vi "Send State.vi"(8 "entrée d'erreur (pas d'erreur)":errorcluster, 11 "State":T1(ring)) -> (0 "sortie d'erreur":errorcluster)   [LabVIEW 2020, in "Library Core.lvlib" / "Actor_EventStart.lvlib" / "Actor_EventStart.lvclass"]
uses:
  Actor_EventStart.lvclass
  Commun VI/TypeDef/Variable Printable.ctl
  Actor_EventStart Messages/Message State/Message State.lvclass/Message State.ctl
  <vilib>/ActorFramework/Message Enqueuer/Message Enqueuer.lvclass/Message Enqueuer.ctl
  <vilib>/ActorFramework/Message Enqueuer/Enqueue.vi
  Actor_EventStart Messages/Message State/Message State.lvclass
  C:/Program Files (x86)/National Instruments/LabVIEW 2020/vi.lib/ActorFramework/Message/Message.lvclass
  <vilib>/ActorFramework/Message Priority Queue/Priority Enqueue.vi
  Commun VI/Library Commun.lvlib
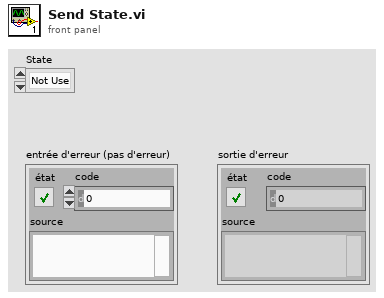
[diagram p1: front panel]
types:
  T1 = enum16{"Not Use", "Wait Event", "Test in progress", "Test Stopped"}
  T2 = enum16{"Get Variable", "Get All Variables", "Set Variable", "Delete Variable", "Delete All Variable"}
  T3 = typedef "Variable Printable.ctl" = string
  T4 = enum16{"Init", "Add Actor", "Delete Actor", "Get Actor Queue", "Get Log Actor Queue", "List all actors"}
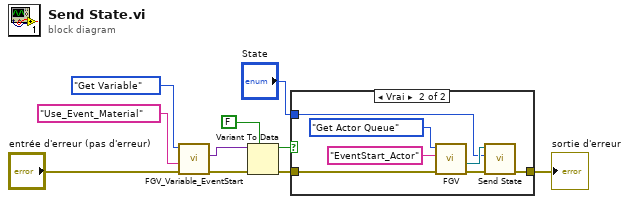
[diagram p0: block diagram]
diagram:
  n1 = call "FGV_Variable_EventStart.vi"("error in (no error)"="entrée d'erreur (pas d'erreur)", "Variable"=T3 "Use_Event_Material", "Function"=T2."Get Variable") -> ("error out"=w3:errorcluster, "Data Out"=w6:variant)  [unwired: 6 in, 1 out]
  n2 = Variant To Data(error in=w3, type=FALSE, Variant=w6) -> (data=w9:bool, error out=w8:errorcluster)
  n3 = case shown="Vrai" w9 {
    tunnel: [w11 w18] -> w1
    tunnel: w8 -> [w11 w17]
    tunnel: "State" -> [_ w12]
    frame False {
    }
    frame True {
      n4 = call "FGV.vi"("error in (no error)"=w17, "Actor name"="EventStart_Actor", "Action"=T4."Get Actor Queue") -> ("error out"=w16:errorcluster, "Actor's Queue Out"=w15:refnum<class "Message Enqueuer.lvclass">)  [unwired: 6 in, 1 out]
      n5 = call "Send State.vi"("error in (no error)"=w16, "State"=w12, "Message Enqueuer"=w15) -> ("error out"=w18:errorcluster)  [unwired: 7 in, 1 out]
    }
  }
  "sortie d'erreur" <- w1
